vi "Main.vi"(11 "Module Admin":refnum<class "Delacor_lib_QMH_Module Admin.lvclass">) -> ()   [LabVIEW 2020, in "Config.lvlib"]
doc: "This template is based off of the Queued Message Handler design pattern and the Queued Message Handler project template that ships with LabVIEW.\n\nThe main difference is that the queue is private to this module and communication between modules is performed via Broadcast and Request events.\n\nRequest events are wrapped in public API methods and are handled in the Event Handling Loop (EHL) of this VI. Any module can register for Broadcast events sent by this module. The EHL generates messages based on user interface actions.\n\nThe Message Handling Loop (MHL) processes messages generated by the EHL, or by other messages. The messages are string values, so new messages can be added easily to the Message Cases case structure in the MHL. Each message cluster can also provide an optional value for Message Data, which is a variant that can be converted to whatever message-specific data is required.\n_____\nBased on Delacor QMH Project Template 5.0.0.82."
uses:
  Config.lvlib
  <vilib>/Delacor/Delacor QMH/Libraries/Module Admin_class/Delacor_lib_QMH_Module Admin.lvclass
  Module Data--cluster.ctl
  Stop Argument--cluster.ctl
  <vilib>/Delacor/Delacor QMH/Libraries/Message Queue_class/Delacor_lib_QMH_Message Queue.lvclass/Delacor_lib_QMH_Message Queue.ctl
  <vilib>/Utility/miscctls.llb/LVPointTypeDef.ctl
  <vilib>/Delacor/Delacor QMH/Libraries/Module Admin_class/Delacor_lib_QMH_Module Admin.lvclass/Delacor_lib_QMH_Module Admin.ctl
  <vilib>/Delacor/Delacor QMH/Libraries/Message Queue_class/Delacor_lib_QMH_Enqueue Message (Single).vi
  <vilib>/Delacor/Delacor QMH/Libraries/Module Admin_class/Delacor_lib_QMH_Get External Launch.vi
  <vilib>/Utility/error.llb/Error Cluster From Error Code.vi
  <vilib>/ErrorRing/Error Ring.xnode
  <vilib>/Delacor/Delacor QMH/Libraries/Message Queue_class/Delacor_lib_QMH_Message Queue.lvclass
  Acquisiton Oscar Template/Acquisiton Oscar Template.lvlib
  Logging/Logging.lvlib
panel:
  in  "phase":dbl
  in  "offset":dbl
  in  "square wave duty cycle (%)":dbl
  in  "amplitude":dbl
  in  "frequency":dbl
  in  "sampling info":cluster{"Fs":dbl, "#s":dbl}
  in  "signal type":T1(ring)
  in  "File Name":string
  out "error out":errorcluster
  out "Status":string
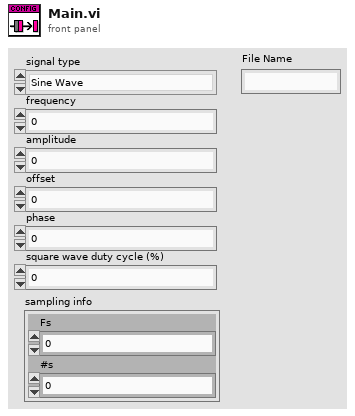
[diagram p1: front panel]
types:
  T1 = enum16{"Sine Wave", "Triangle Wave", "Square Wave", "Sawtooth Wave"}
  T2 = typedef "Config.lvlib/Request Events--cluster.ctl" = cluster{"Stop Module":refnum<user-event>, "Show Panel":refnum<user-event>, "Hide Panel":refnum<user-event>, "Get Module Execution Status":refnum<user-event>, "Show Diagram":refnum<user-event>}
  T3 = typedef "Config.lvlib/Module Data--cluster.ctl" = cluster{"Status":string}
  T4 = enum32{"invalid lock state", "Not Locked", "Locked (No Password)", "Password-protected"}
  T5 = typedef "Config.lvlib/Stop Argument--cluster.ctl" = cluster{"Origin":string, "Exit via Stop Module Req?":bool, "Wait for Module to stop?":bool}
  T6 = cluster{"signal type":enum16{"Sine Wave", "Triangle Wave", "Square Wave", "Sawtooth Wave"}, "sampling info":cluster{"Fs":dbl, "#s":dbl}, "frequency":dbl, "amplitude":dbl, "square wave duty cycle (%)":dbl, "offset":dbl, "phase":dbl}
  T7 = typedef "LVPointTypeDef.ctl" = cluster{"Horizontal":i16, "Vertical":i16}
  T8 = enum32{"Invalid", "Standard", "Closed", "Hidden", "Minimized", "Maximized"}
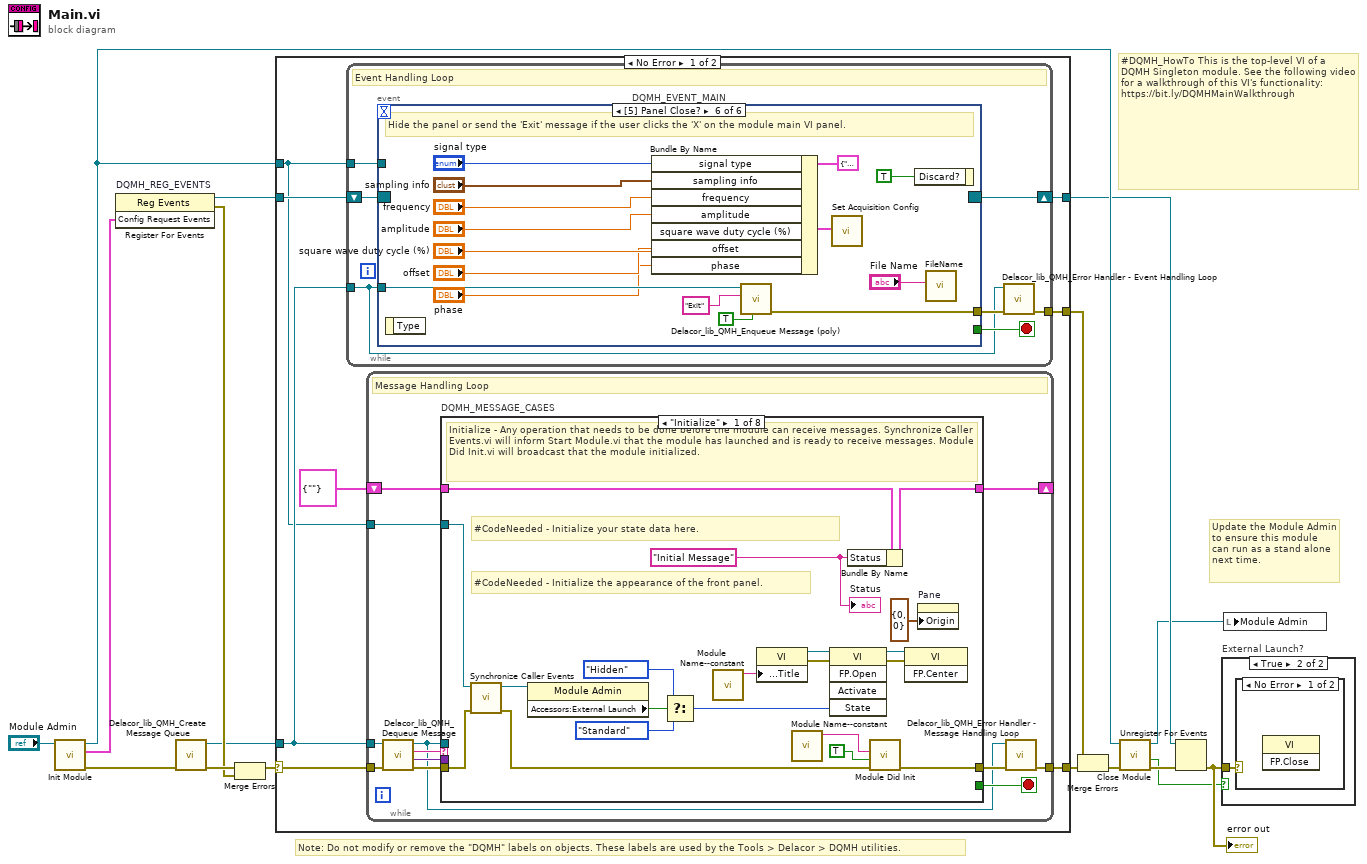
[diagram p0: block diagram]
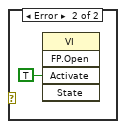
[diagram p3: hidden frame]
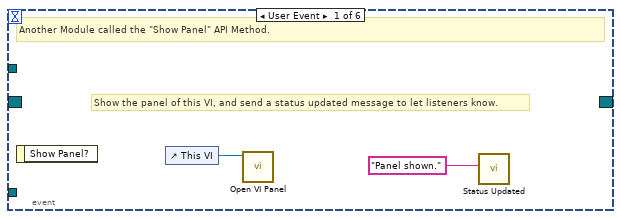
[diagram p4: hidden frame]
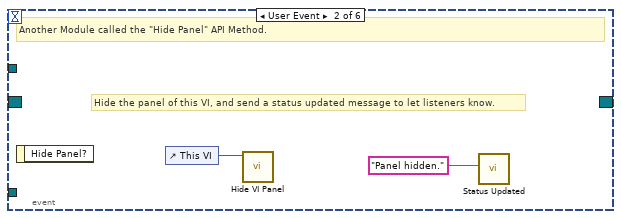
[diagram p5: hidden frame]
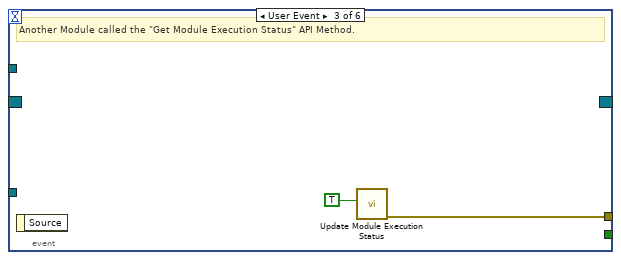
[diagram p6: hidden frame]
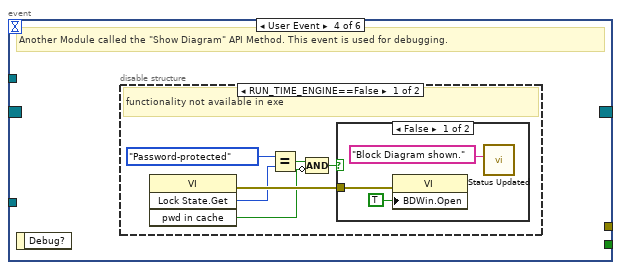
[diagram p7: hidden frame]
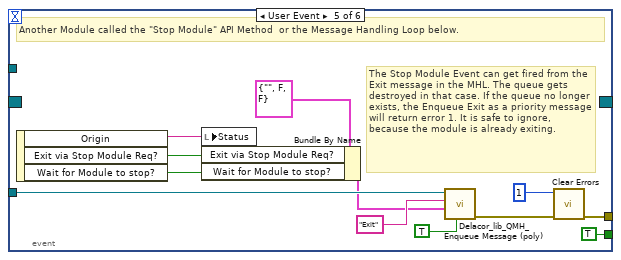
[diagram p10: hidden frame]
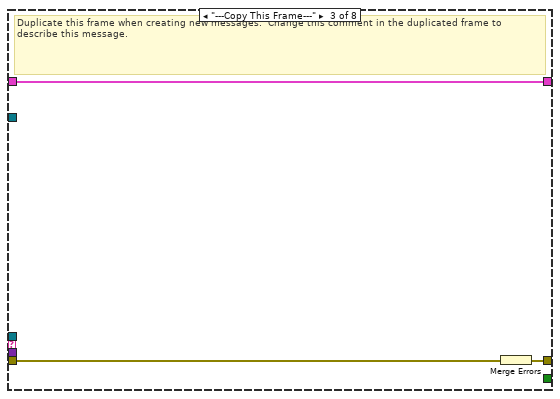
[diagram p12: hidden frame]
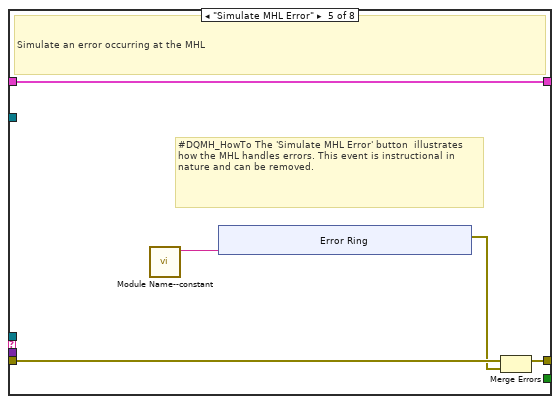
[diagram p14: hidden frame]
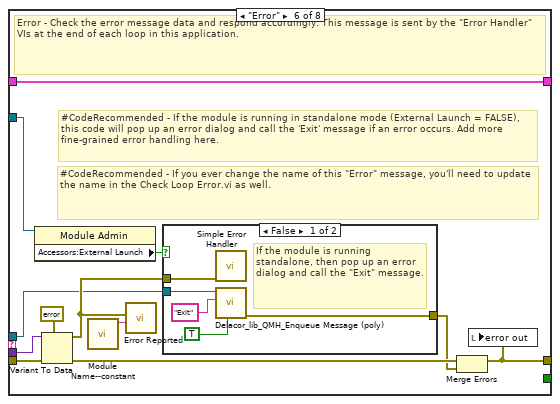
[diagram p15: hidden frame]
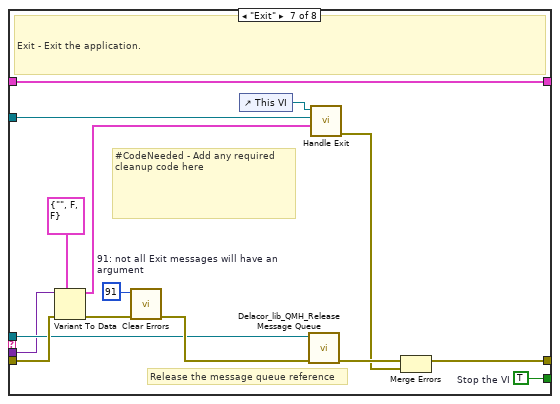
[diagram p17: hidden frame]
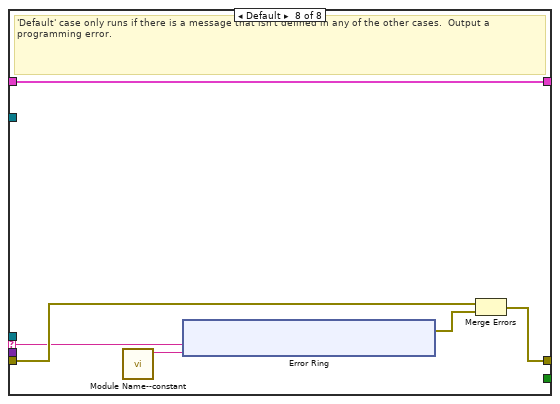
[diagram p18: hidden frame]
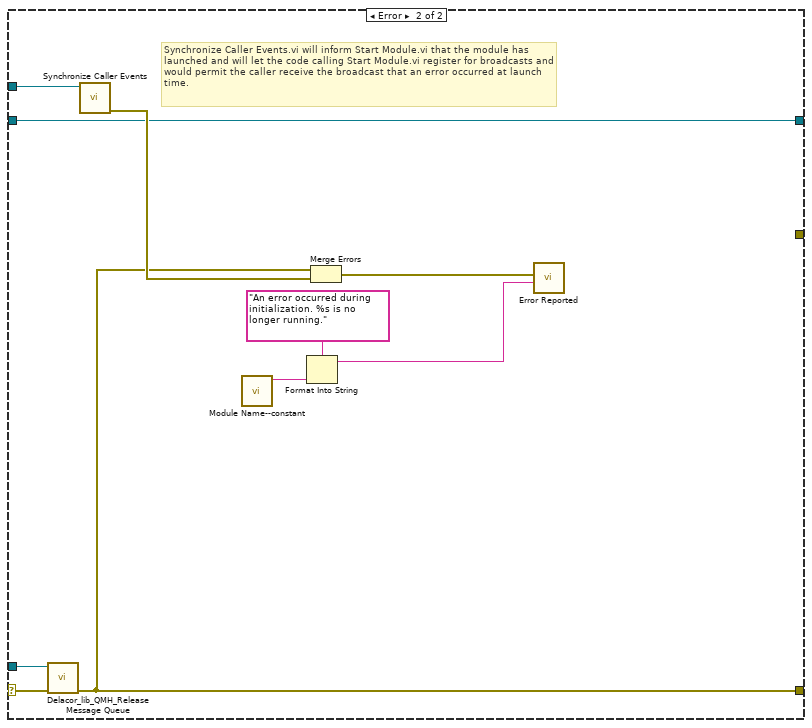
[diagram p19: hidden frame]
diagram:
  # "#DQMH_HowTo This is the top-level VI of a DQMH Singleton module. See the following video for a walkthrough of this VI's functionality: https://bit.ly/DQMHMainWalkthrough"
  # "Note: Do not modify or remove the \"DQMH\" labels on objects. These labels are used by the Tools > Delacor > DQMH utilities."
  # "Update the Module Admin to ensure this module can run as a stand alone next time."
  n1 = call "Init Module.vi"("Singleton Module Admin in"="Module Admin") -> ("error out"=w16:errorcluster, "Config Request Events"=w5:T2, "Singleton Module Admin out"=w8:refnum<class "Delacor_lib_QMH_Module Admin.lvclass">)  [unwired: 8 in]
  n2 = register-events "DQMH_REG_EVENTS"(w5) -> (reference out=w6:refnum<event-registration>, error out=w9:errorcluster)  [unwired: 2 in]
  n3 = call <vilib>:"Delacor_lib_QMH_Create Message Queue.vi"("error in (no error)"=w16) -> ("error out"=w11:errorcluster, "Message Queue"=w4:refnum<class "Delacor_lib_QMH_Message Queue.lvclass">)  [unwired: 9 in]
  n4 = Merge Errors(w11, w9) -> (w10:errorcluster)
  n5 = case shown="No Error" w10 {
    selector: w10 -> [w23 w174]
    tunnel: [w25 w173] -> w17
    tunnel: [w22 w179] -> w7
    tunnel: w6 -> [w20 w179]
    tunnel: w4 -> [w19 w172]
    tunnel: [w24 _] -> w14
    tunnel: w8 -> [w18 w175]
    frame No Error {
      n6 = while {
        tunnel: w19 -> [w26]
        shift-right: [w29] -> w22
        shift-left: w20 -> [w30]
        tunnel: [w31] -> w24
        tunnel: w18 -> [w27]
        stop <- w28 stop-if-true
        # "Event Handling Loop"
        n7 = event "DQMH_EVENT_MAIN" shown="[5] Panel Close?" {
          selector: w30 -> [_ _ _ _ _ _]
          dyn-events: [_ _ _ _ _ _] -> w29
          timeout: _ -> [_ _ _ _ _ _]
          tunnel: [_ _ _ _ TRUE ("Discard?") _] -> w28
          tunnel: w26 -> [_ _ _ _ w55 w72]
          tunnel: [_ _ w38 _ w58 w74] -> w32
          tunnel: w27 -> [_ _ _ _ _ _]
          event User Event {
            # "Show the panel of this VI, and send a status updated message to let listeners know."
            # "Another Module called the \"Show Panel\" API Method."
            n8 = event-data() -> ()  [unwired: 1 in, 1 out]
            n9 = control-ref of="This VI"() -> (w34:refnum<vi>)
            n10 = call "Open VI Panel.vi"("VI"=w34) -> ()  [unwired: 10 in, 1 out]
            n11 = call "Status Updated.vi"("Status"="Panel shown." ("format string")) -> ()  [unwired: 10 in, 1 out]
          }
          event User Event {
            # "Hide the panel of this VI, and send a status updated message to let listeners know."
            # "Another Module called the \"Hide Panel\" API Method."
            n12 = event-data() -> ()  [unwired: 1 in, 1 out]
            n13 = control-ref of="This VI"() -> (w36:refnum<vi>)
            n14 = call "Hide VI Panel.vi"("VI"=w36) -> ()  [unwired: 10 in, 1 out]
            n15 = call "Status Updated.vi"("Status"="Panel hidden." ("format string")) -> ()  [unwired: 10 in, 1 out]
          }
          event User Event {
            # "Another Module called the \"Get Module Execution Status\" API Method."
            n16 = event-data() -> ()  [unwired: 1 in, 1 out]
            n17 = call "Update Module Execution Status.vi"("Running?"=TRUE) -> ("error out"=w38:errorcluster)  [unwired: 10 in]
          }
          event User Event {
            # "Another Module called the \"Show Diagram\" API Method. This event is used for debugging."
            n18 = event-data() -> ()  [unwired: 1 in, 1 out]
            n19 = disable-structure shown="RUN_TIME_ENGINE==False" {
              frame condition #0 (active) {
                # "functionality not available in exe"
                n20 = invoke class="VI" method="Lock State.Get"() -> (error out=w44:errorcluster, "Get Lock State"=w43:T4, "pwd in cache"=w40:bool)  [unwired: 4 in, 1 out]
                n21 = Equal?(x=T4."Password-protected", y=w43) -> (x = y?=w41:bool)
                n22 = Compound Arithmetic op=AND(w41, invert w40) -> (w39:bool)
                n23 = case shown="False" w39 {
                  tunnel: w44 -> [w47 _]
                  frame False {
                    n24 = property class="VI"(error in=w47, "BDWin.Open"=TRUE ("Block Diagram Window:Open")) -> ()  [unwired: 1 in, 2 out]
                    n25 = call "Status Updated.vi"("Status"="Block Diagram shown." ("format string")) -> ()  [unwired: 10 in, 1 out]
                  }
                  frame True {
                    # "Password-protected VI, and the password is not in the cache. Do not show the diagram."
                  }
                }
              }
              frame condition #1 {
              }
            }
          }
          event User Event {
            # "The Stop Module Event can get fired from the Exit message in the MHL. The queue gets destroyed in that case. If the queue no longer exists, the Enqueue Exit as a priority message will return error 1. It is safe to ignore, because the module is already exiting."
            # "Another Module called the \"Stop Module\" API Method  or the Message Handling Loop below."
            n26 = event-data() -> ("Origin"=w54:string, "Exit via Stop Module Req?"=w50:bool, "Wait for Module to stop?"=w49:bool)  [unwired: 1 in]
            n27 = local write "Status"(w54) -> ()
            n28 = Bundle By Name(cluster=T5 {"Origin"="", "Exit via Stop Module Req?"=FALSE, "Wait for Module to stop?"=FALSE} ("Stop Argument"), "Exit via Stop Module Req?"=w50, "Wait for Module to stop?"=w49) -> (w48:T5)
            n29 = call-poly <vilib>:"Delacor_lib_QMH_Enqueue Message (poly).vi"("Priority Message? (F)"=TRUE, "Message Data"=w48, "Message"="Exit", "Message Queue in"=w55) -> ("error out"=w59:errorcluster)  [unwired: 6 in, 1 out]
            n30 = call <vilib>:"Clear Errors.vi"("error in (no error)"=w59, "specific error code to clear (0: all)"=1) -> ("error out"=w58:errorcluster)  [unwired: 4 in, 1 out]
          }
          event Panel Close? {
            # "Hide the panel or send the 'Exit' message if the user clicks the 'X' on the module main VI panel."
            n31 = event-data() -> ()  [unwired: 1 in, 1 out]
            n32 = Bundle By Name(cluster=T6 {"signal type"=enum."Sine Wave", "sampling info"={"Fs"=1000.0, "#s"=1000.0}, "frequency"=10.0, "amplitude"=1.0, "square wave duty cycle (%)"=50.0, "offset"=0.0, "phase"=0.0} ("Cluster"), "signal type"="signal type", "sampling info"="sampling info", "frequency"="frequency", "amplitude"="amplitude", "square wave duty cycle (%)"="square wave duty cycle (%)", "offset"="offset", "phase"="phase") -> (w67:T6)
            n33 = call-poly <vilib>:"Delacor_lib_QMH_Enqueue Message (poly).vi"("Priority Message? (F)"=TRUE, "Message"="Exit", "Message Queue in"=w72) -> ("error out"=w74:errorcluster)  [unwired: 7 in, 1 out]
            n34 = call "Set Acquisition Config.vi"("Cluster"=w67) -> ()  [unwired: 10 in, 1 out]
            n35 = event-data("Discard?"=TRUE ("Discard the event, the MHL is responsible for closing and stopping this VI.")) -> ()  [unwired: 1 in, 1 out]
            n36 = call "FileName.vi"("File Name"="File Name") -> ()  [unwired: 10 in, 1 out]
          }
        }
        n37 = call-dynamic "Delacor_lib_QMH_Error Handler - Event Handling Loop.vi"("error in (no error)"=w32, "Message Queue in"=w26) -> ("dup error in"=w31:errorcluster)  [unwired: 8 in, 1 out]
      }
      n38 = while {
        tunnel: w19 -> [w77]
        shift-right: [w81] -> _
        shift-left: T3 {"Status"=""} ("Data Cluster") -> [w82]
        tunnel: w23 -> [w85]
        tunnel: [w83] -> w25
        tunnel: w18 -> [w75]
        stop <- w80 stop-if-true
        # "Message Handling Loop"
        n39 = call-dynamic "Delacor_lib_QMH_Dequeue Message.vi"("error in (no error)"=w85, "Message Queue in"=w77) -> ("error out"=w84:errorcluster, "Message Data"=w78:variant, "Message"=w79:string, "Message Queue out"=w76:refnum<class "Delacor_lib_QMH_Message Queue.lvclass">)  [unwired: 6 in]
        n40 = case "DQMH_MESSAGE_CASES" shown="\"Initialize\"" w79 {
          selector: w79 -> [_ _ _ _ _ _ _ w159]
          tunnel: w76 -> [_ _ _ _ _ w129 w151 _]
          tunnel: w84 -> [w104 w108 w111 w113 w118 w136 w157 w161]
          tunnel: [w102 w108 w110 w113 w117 w132 w154 w162] -> w86
          tunnel: w82 -> [w93 w107 w109 w112 w115 w131 w150 w160]
          tunnel: [w92 w107 w109 w112 w115 w131 w150 w160] -> w81
          tunnel: [_ _ _ _ _ _ w149 _] -> w80
          tunnel: w78 -> [_ _ _ _ _ w130 w148 _]
          tunnel: w75 -> [w94 _ _ _ _ w128 w143 _]
          frame "Initialize" {
            w87 = "Initial Message" ("Initial Message")
            # "#CodeNeeded - Initialize the appearance of the front panel."
            # "#CodeNeeded - Initialize your state data here."
            # "Initialize - Any operation that needs to be done before the module can receive messages. Synchronize Caller Events.vi will inform Start Module.vi that the module has launched and is ready to receive messages. Module Did Init.vi will broadcast that the module initialized."
            n41 = call "Synchronize Caller Events.vi"("error in (no error)"=w104, "Singleton Module Admin in"=w94) -> ("error out"=w103:errorcluster, "Singleton Module Admin out"=w89:refnum<class "Delacor_lib_QMH_Module Admin.lvclass">)  [unwired: 8 in]
            n42 = property class="Module Admin"(reference=w89) -> ("Accessors:External Launch"=w98:bool)  [unwired: 1 in, 2 out]
            n43 = Select(t=T8."Hidden" ("State"), s=w98, f=T8."Standard" ("State")) -> (s? t:f=w95:T8)
            n44 = call "Module Name--constant.vi"() -> ("Module Name"=w101:string)  [unwired: 11 in]
            n45 = property class="VI"("Front Panel.Title"=w101) -> (reference out=w100:refnum<vi>, error out=w106:errorcluster)  [unwired: 2 in]
            n46 = call "Module Name--constant.vi"() -> ("Module Name"=w90:string)  [unwired: 11 in]
            n47 = invoke class="VI" method="FP.Open"(reference=w100, error in=w106, "State"=w95) -> (reference out=w99:refnum<vi>, error out=w105:errorcluster)  [unwired: 2 in, 3 out]
            n48 = Bundle By Name(cluster=w93, "Status"=w87) -> (w92:T3)
            n49 = call "Module Did Init.vi"("error in (no error)"=w103, "Initialized?"=TRUE, "Origin"=w90) -> ("error out"=w102:errorcluster)  [unwired: 8 in]
            n50 = invoke class="VI" method="FP.Center"(reference=w99, error in=w105) -> ()  [unwired: 1 in, 3 out]
            n51 = property on="Pane" class="Pane"("Origin"=T7 {"Horizontal"=0, "Vertical"=0}) -> ()  [unwired: 2 in, 2 out]
            "Status" <- w87
          }
          frame "--- Module Specific ---" {
            # "Separator -- The following cases handle messages specific to this Module."
          }
          frame "---Copy This Frame---" {
            # "Duplicate this frame when creating new messages.  Change this comment in the duplicated frame to describe this message."
            n52 = Merge Errors(w111) -> (w110:errorcluster)
          }
          frame "--- Exit and Error Handling---" {
            # "Separator - The following cases handle errors and exit messages."
          }
          frame "Simulate MHL Error" {
            # "#DQMH_HowTo The 'Simulate MHL Error' button  illustrates how the MHL handles errors. This event is instructional in nature and can be removed."
            # "Simulate an error occurring at the MHL"
            n53 = call "Module Name--constant.vi"() -> ("Module Name"=w114:string)  [unwired: 11 in]
            n54 = xnode "Error Ring"("parameter 0"=w114) -> ("error out"=w116:errorcluster)
            n55 = Merge Errors(w118, w116) -> (w117:errorcluster)
          }
          frame "Error" {
            # "#CodeRecommended - If you ever change the name of this \"Error\" message, you'll need to update the name in the Check Loop Error.vi as well."
            # "#CodeRecommended - If the module is running in standalone mode (External Launch = FALSE), this code will pop up an error dialog and call the 'Exit' message if an error occurs. Add more fine-grained error handling here."
            # "Error - Check the error message data and respond accordingly. This message is sent by the \"Error Handler\" VIs at the end of each loop in this application."
            n56 = property class="Module Admin"(reference=w128) -> ("Accessors:External Launch"=w127:bool)  [unwired: 1 in, 2 out]
            n57 = Variant To Data(error in=w136, type=errorcluster {"status"=FALSE, "code"=0, "source"=""} ("error constant"), Variant=w130) -> (data=w137:errorcluster, error out=w134:errorcluster)
            n58 = call "Module Name--constant.vi"() -> ("Module Name"=w126:string)  [unwired: 11 in]
            n59 = call "Error Reported.vi"("Additional Information"=w126, "Error"=w137) -> ()  [unwired: 9 in, 1 out]
            n60 = case shown="False" w127 {
              tunnel: [w142 _] -> w133
              tunnel: w129 -> [w140 _]
              tunnel: w137 -> [w141 _]
              frame False {
                # "If the module is running standalone, then pop up an error dialog and call the \"Exit\" message."
                n61 = call <vilib>:"Simple Error Handler.vi"("error in (no error)"=w141) -> ()  [unwired: 4 in, 5 out]
                n62 = call-poly <vilib>:"Delacor_lib_QMH_Enqueue Message (poly).vi"("Priority Message? (F)"=TRUE, "Message"="Exit", "Message Queue in"=w140) -> ("error out"=w142:errorcluster)  [unwired: 7 in, 1 out]
              }
              frame True {
                # "If the module was launched externally, calling the Error Reported broadcast VI is the only action performed by the \"Error\" message. The module's caller can then process the error appropriately."
              }
            }
            n63 = Merge Errors(w134, w133) -> (w132:errorcluster)
            n64 = local write "error out"(w132) -> ()
          }
          frame "Exit" {
            w147 = 91  # 91: not all Exit messages will have an argument
            w149 = TRUE  # Stop the VI
            # "Release the message queue reference"
            # "#CodeNeeded - Add any required cleanup code here"
            # "Exit - Exit the application."
            n65 = Variant To Data(error in=w157, type=T5 {"Origin"="", "Exit via Stop Module Req?"=FALSE, "Wait for Module to stop?"=FALSE} ("Stop Argument"), Variant=w148) -> (data=w145:T5, error out=w153:errorcluster)
            n66 = call <vilib>:"Clear Errors.vi"("error in (no error)"=w153, "specific error code to clear (0: all)"=w147) -> ("error out"=w156:errorcluster)  [unwired: 4 in, 1 out]
            n67 = control-ref of="This VI"() -> (w144:refnum<vi>)
            n68 = call-dynamic "Delacor_lib_QMH_Release Message Queue.vi"("error in (no error)"=w156, "Message Queue"=w151) -> ("error out"=w155:errorcluster)  [unwired: 9 in]
            n69 = call "Handle Exit.vi"("Stop Argument"=w145, "Admin in"=w143, "VI reference"=w144) -> ("error out"=w152:errorcluster)  [unwired: 7 in, 1 out]
            n70 = Merge Errors(w155, w152) -> (w154:errorcluster)
          }
          frame Default {
            # "'Default' case only runs if there is a message that isn't defined in any of the other cases.  Output a programming error."
            n71 = call "Module Name--constant.vi"() -> ("Module Name"=w158:string)  [unwired: 11 in]
            n72 = xnode "Error Ring"("parameter 0"=w159, "parameter 1"=w158) -> ("error out"=w163:errorcluster)
            n73 = Merge Errors(w161, w163) -> (w162:errorcluster)
          }
        }
        n74 = call-dynamic "Delacor_lib_QMH_Error Handler - Message Handling Loop.vi"("error in (no error)"=w86, "Message Queue in"=w76) -> ("dup error in"=w83:errorcluster)  [unwired: 8 in, 1 out]
      }
    }
    frame Error {
      # "Synchronize Caller Events.vi will inform Start Module.vi that the module has launched and will let the code calling Start Module.vi register for broadcasts and would permit the caller receive the broadcast that an error occurred at launch time."
      n75 = call-dynamic "Delacor_lib_QMH_Release Message Queue.vi"("error in (no error)"=w174, "Message Queue"=w172) -> ("error out"=w173:errorcluster)  [unwired: 9 in]
      n76 = call "Synchronize Caller Events.vi"("Singleton Module Admin in"=w175) -> ("error out"=w180:errorcluster)  [unwired: 9 in, 1 out]
      n77 = call "Module Name--constant.vi"() -> ("Module Name"=w178:string)  [unwired: 11 in]
      n78 = Format Into String(format string="An error occurred during initialization. %s is no longer running.", w178) -> (resulting string=w176:string)  [unwired: 2 in, 1 out]
      n79 = Merge Errors(w173, w180) -> (w181:errorcluster)
      n80 = call "Error Reported.vi"("Additional Information"=w176, "Error"=w181) -> ()  [unwired: 9 in, 1 out]
    }
  }
  n81 = Merge Errors(w14, w17) -> (w13:errorcluster)
  n82 = call "Close Module.vi"("error in (no error)"=w13, "Module Admin in"=w8) -> ("error out"=w15:errorcluster, "External Launch"=w1:bool, "Module Admin out"=w2:refnum<class "Delacor_lib_QMH_Module Admin.lvclass">)  [unwired: 7 in]
  n83 = Unregister For Events(event registration refnum=w7, error in=w15) -> (error out=w12:errorcluster)
  "error out" <- w12
  n84 = case "External Launch?" shown="True" w1 {
    tunnel: w12 -> [_ w182]
    frame False {
    }
    frame True {
      n85 = case shown="No Error" w182 {
        frame No Error {
          n86 = invoke class="VI" method="FP.Close"() -> ()  [unwired: 3 in, 3 out]
        }
        frame Error {
          n87 = invoke class="VI" method="FP.Open"("Activate"=TRUE ("Activate?")) -> ()  [unwired: 4 in, 5 out]
        }
      }
    }
  }
  n88 = local write "Module Admin"(w2) -> ()
